vi "File Naming From Selection.vi"(0 "Subject In":string, 5 "Test Type In":T1 items=["Practice Trials", "Mechanical (Mask)", "Mechanical (Mouthpiece)", "Labial (Normal)", "Labial (Quiet)"], 11 "Error In":errorcluster) -> (4 "File Name":string, 6 "Test Type":string, 8 "Delay":u32, 10 "Interruptions":u32, 15 "Error Out":errorcluster)   [LabVIEW 2013, in "CollectionSupport.lvlib"]
uses:
  CollectionSupport.lvlib
  Controls/Mech-Labial Test Types.ctl
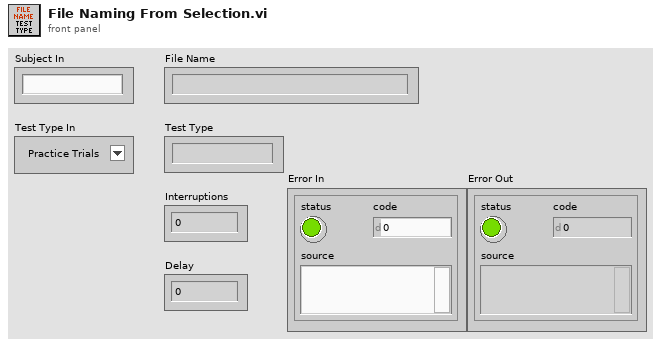
[diagram p1: front panel]
types:
  T1 = typedef "CollectionSupport.lvlib/Mech-Labial Test Types.ctl" = u16
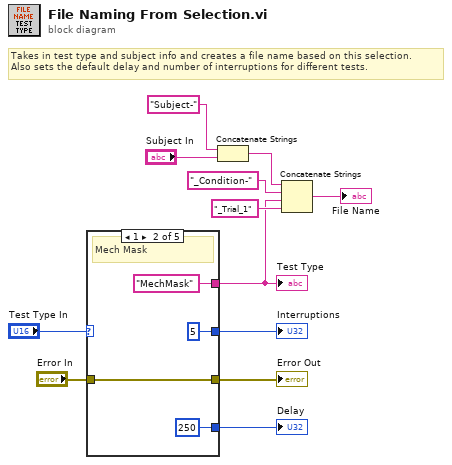
[diagram p0: block diagram]
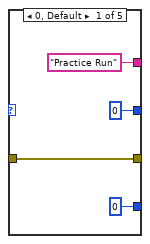
[diagram p2: hidden frame]
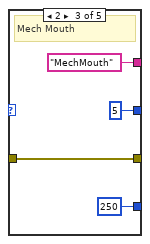
[diagram p3: hidden frame]
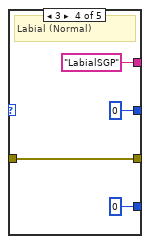
[diagram p4: hidden frame]
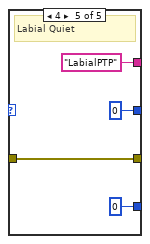
[diagram p5: hidden frame]
diagram:
  # "Takes in test type and subject info and creates a file name based on this selection. \nAlso sets the default delay and number of interruptions for different tests."
  n1 = case shown="1" "Test Type In" {
    tunnel: ["Practice Run" ("string") "MechMask" ("string") "MechMouth" ("string") "LabialSGP" ("string") "LabialPTP" ("string")] -> w4
    tunnel: [u32 0 ("Delay") u32 250 ("Delay") u32 250 ("Delay") u32 0 ("Delay") u32 0 ("Delay")] -> w11
    tunnel: [0 ("Interruptions") u32 5 ("Delay") u32 5 ("Delay") u32 0 ("Delay") u32 0 ("Delay")] -> w12
    tunnel: [w13 w17 w21 w25 w29] -> w2
    tunnel: "Error In" -> [w13 w17 w21 w25 w29]
    frame 0, Default {
    }
    frame 1 {
      # "Mech Mask"
    }
    frame 2 {
      # "Mech Mouth"
    }
    frame 3 {
      # "Labial (Normal)"
    }
    frame 4 {
      # "Labial Quiet"
    }
  }
  "Interruptions" <- w12
  "Delay" <- w11
  "Test Type" <- w4
  "Error Out" <- w2
  n2 = Concatenate Strings("Subject-" ("default name"), "Subject In") -> (w8:string)
  n3 = Concatenate Strings(w8, "_Condition-" ("string"), w4, "_Trial_1" ("string")) -> (→"File Name":string)
